vi "DASDevel.vi"() -> ()   [LabVIEW 2012]
uses:
  <vilib>/Utility/error.llb/DialogType.ctl
  SITK/Documents/SIToolkit/LabVIEW/Examples2012_4_1_0_4/Open-Close/CamHandle.vi
panel:
  out "Database OK?":bool
  in  "?":bool
  in  "Cycle Devices (Red)\nAcquisition (Blue)":bool
  in  "Image Tabs":T1(tab)
  in  "Display Image":dbl(ring) items=["2014-01-09_18;19;45", "2014-01-09_18;20;17"]
  out "Normalized Image":dbl[][](graph)
  out "Atoms":i16[][](graph)
  out "No Atoms":i16[][](graph)
  out "Dark Field":i16[][](graph)
  in  "Image Tabs 2":T1(tab)
  out "Intensity Graph":dbl[][](graph)
  out "PF Atoms":u16[][](graph)
  out "PF No Atoms":u16[][](graph)
  out "PF Dark":u16[][](graph)
  in  "Record 3":bool
  in  "bUseBuffer1 3":bool
  in  "bUseBuffer0 3":bool
  in  "Record 2":bool
  in  "bUseBuffer1 2":bool
  in  "bUseBuffer0 2":bool
  in  "bUseBuffer0":bool
  in  "bUseBuffer1":bool
  in  "Open StructureIn":T2={"Size"=88, "InterfaceType"=0, "Camera Number"=0, "CameraNumAtInterface"=0, "OpenFlags"=[], "OpenDWFlags"=[], "OpenPtrs"=[]}
  out "Bits/pixel":u16
  out "BufNr1":i16
  out "BufNr0":i16
  in  "error in (no error)":errorcluster
  in  "Camera Handle 2":u32
  in  "File and Display Name 2":string
  in  "error in (no error) 2":errorcluster
  in  "Errors":errorcluster
  in  "?":T3(tab)
  in  "Scaling":dbl(slide)=0.0016108638057548662 scale=0.001..0.1
  in  "PF Scale":dbl(slide)=0.9838778342396336 scale=0.001..10.0
  out "Elapsed Time":u32
  out "Database Output":string
  in  "ADC Gain":i32=-1 min=-1 step=1
  in  "ADC Speed":i32=-1 min=-3 step=1
  in  "Exposure (sec)":dbl format="%.3f"
  in  "Number of Images":u32=1
  in  "Number of Accumulations":u32=1
  in  "Acquire / Focus Flag":u32(ring)=2 items=["Synchronous Focus Mode"=1, "Synchronous NFrame Mode"=2, "Asynchronous Mode"=3, "Sequence Mode"=4]
  in  "Timing Mode":u32(ring)=4 items=["Free Run"=1, "Trigger First"=2, "Strobe"=3, "Bulb"=4, "Variable"=5, "Flash"=6]
  in  "Trigger Edge":u32(ring)=1 items=["Rising"=1, "Falling"=2]
  in  "Milliseconds Between Shots":u32=200
  in  "TriggerMode":u16(ring)=2 items=["Auto", "Software", "External sequence start ", "External exposure control"]
  in  "StorageMode":bool
  in  "Delay":u32=100
  in  "Exposure":u32=30
  in  "ExposureTimeBase":u16(ring)=1 items=["nanoseconds", "microseconds", "milliseconds"]
  in  "DelayTimeBase":u16(ring)=2 items=["nanoseconds", "microseconds", "milliseconds"]
  in  "ROIX0":u16=1 min=1
  in  "ROIY0":u16=1 min=1
  in  "ROIY1":u16=1 min=1
  in  "ROIX1":u16=1 min=1
  in  "Rate":i32
  in  "InterfaceType":u16(ring)=6 items=["IEEE1394 - Firewire", "IEEE1394/Firewire", "Matrox Helios Camera Link", "Silicon Software ME3 Camera Link", "National Instruments Camera Link", "Gigabit Ethernet", "USB", "Reserved", "Reserved", "Reserved", "Generic Camera Link with CLSER.DLL"]
  out "Top of Chamber Monitor":dynamicdata(graph)
  # "Stop Button"
  # "DAS Mode Select"
  # "CoolSnap HQ"
  # "PixelFly"
  # "Basic Setup"
  # "Triggering Setup"
  # "Advanced Setup"
  # "For everyday use, Number of Accumulations should be 1"
  # "Basic Setup for PixelFly"
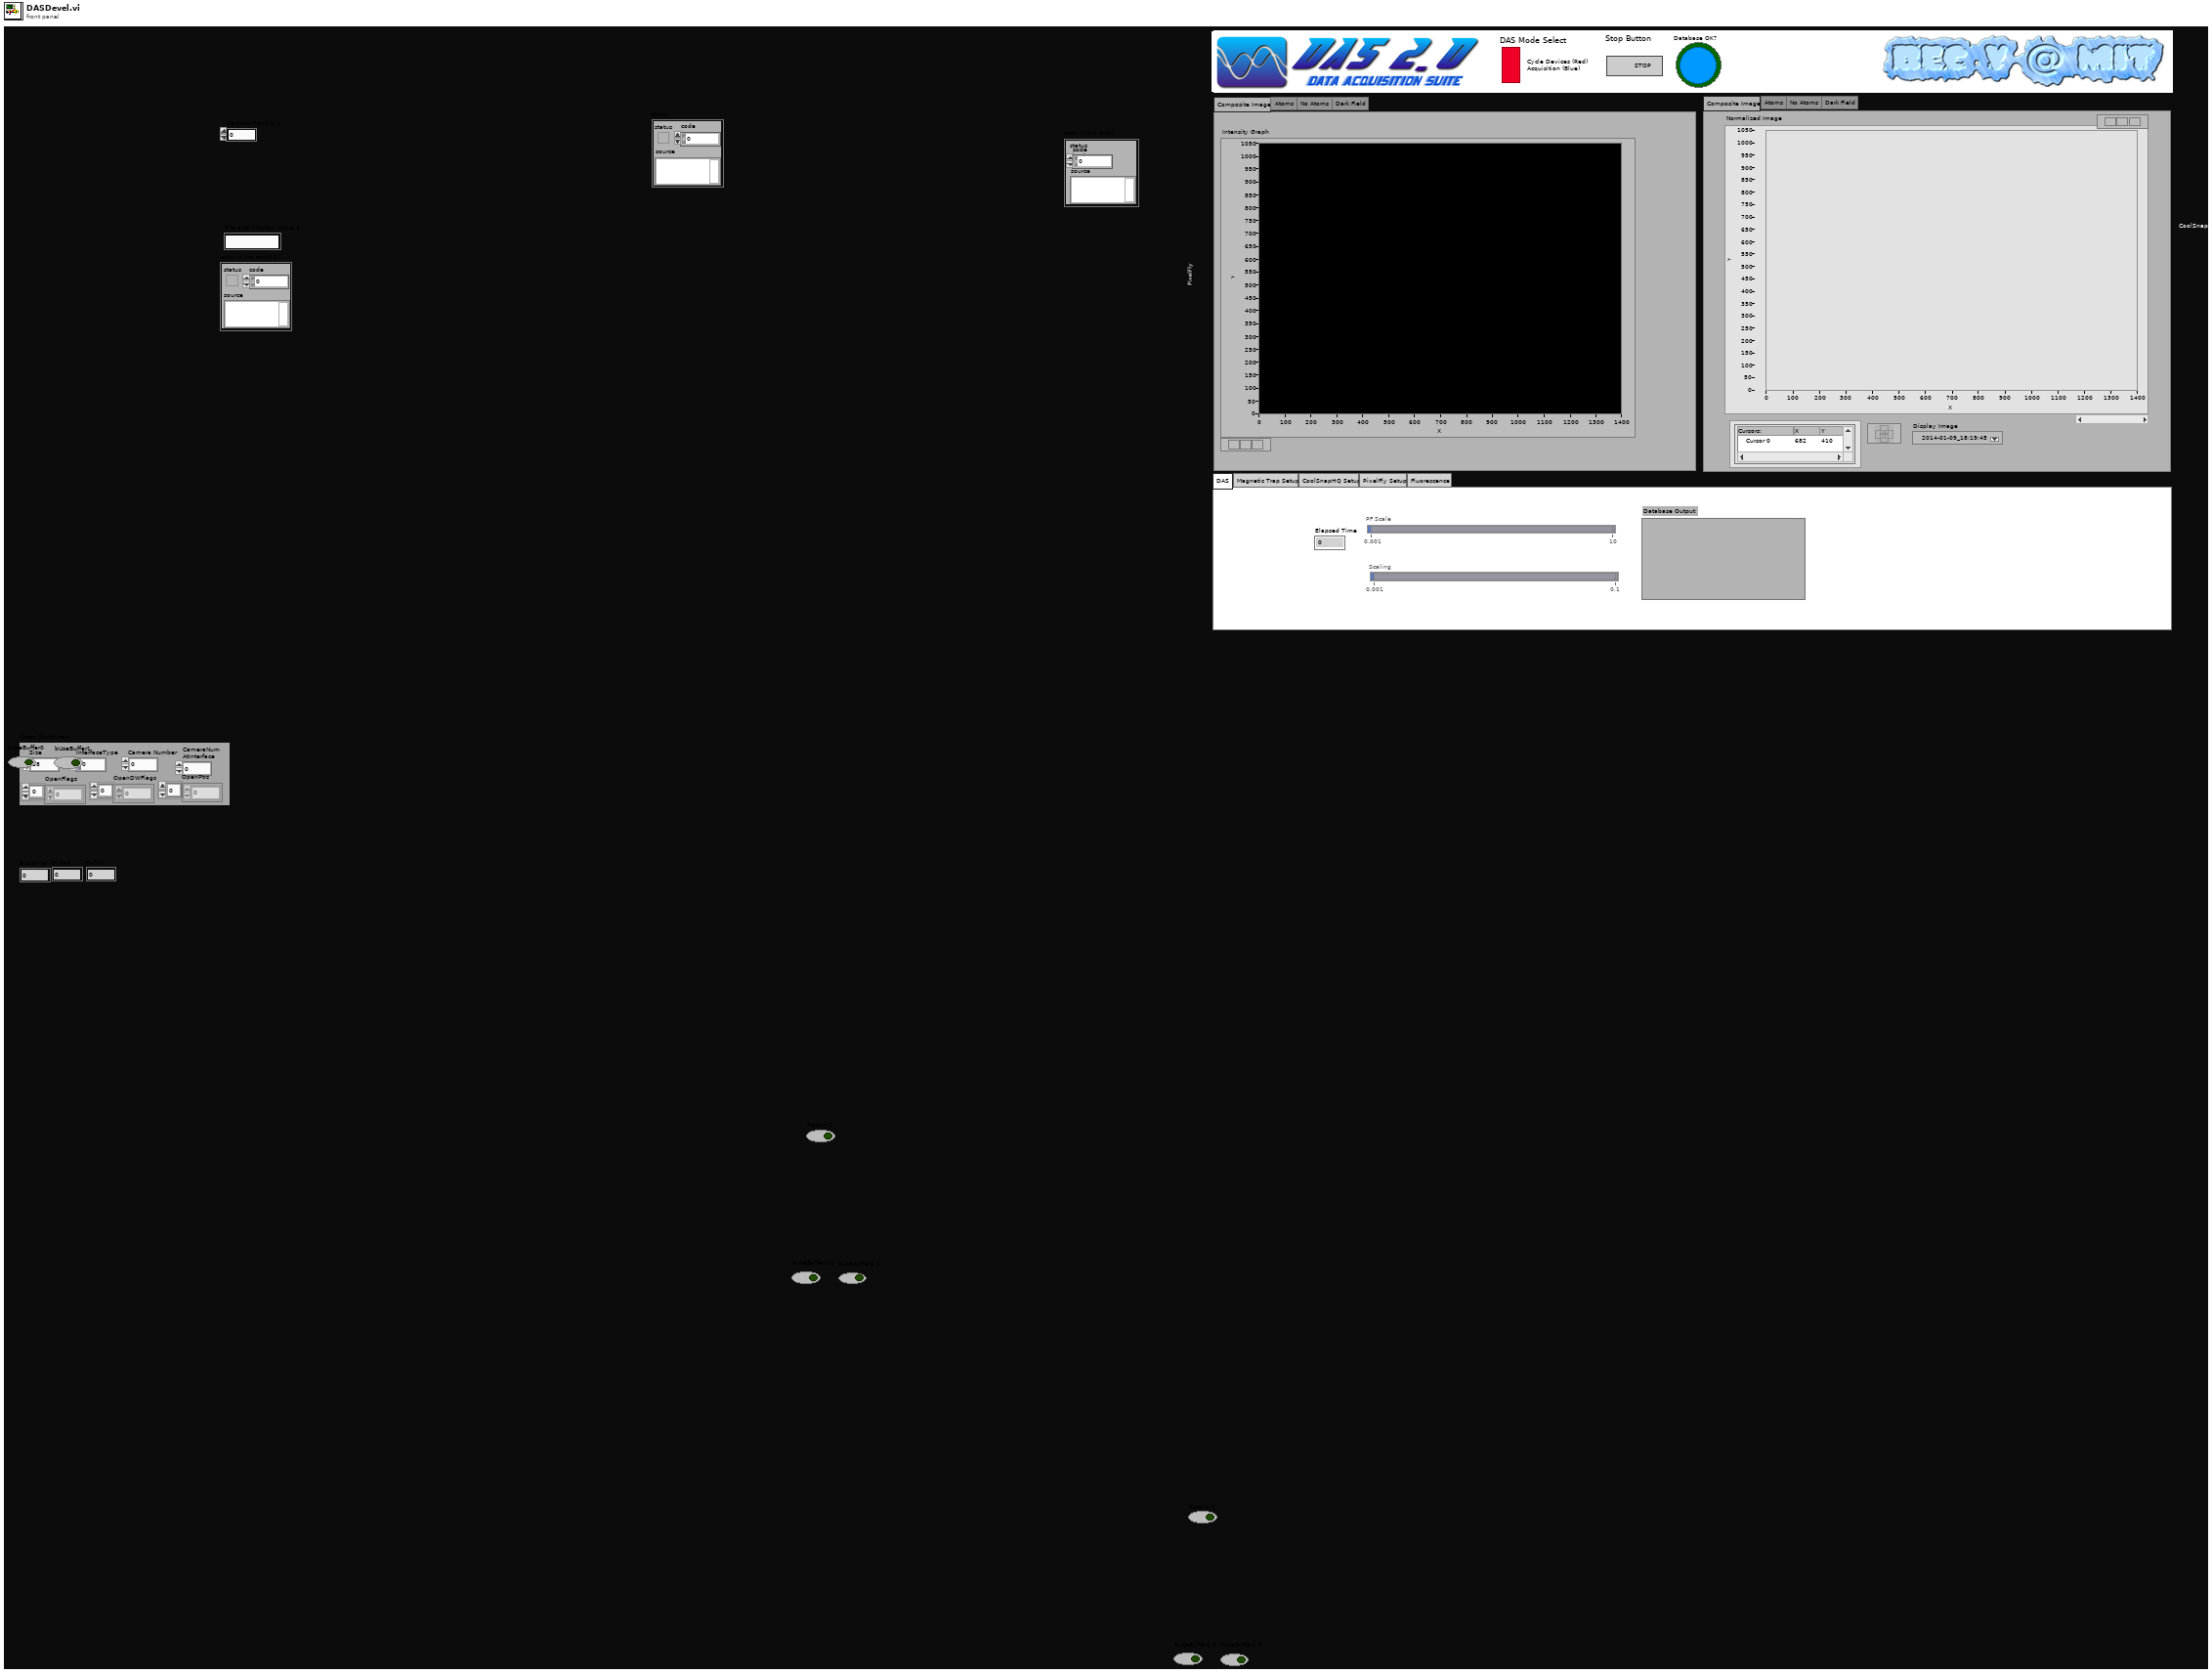
[diagram p1: front panel]
types:
  T1 = enum32{"Composite Image", "Atoms", "No Atoms", "Dark Field"}
  T2 = cluster{"Size":u16, "InterfaceType":u16, "Camera Number":u16, "CameraNumAtInterface":u16, "OpenFlags":u16[], "OpenDWFlags":u32[], "OpenPtrs":u32[]}
  T3 = enum32{"DAS", "Magnetic Trap Setup", "CoolSnapHQ Setup", "PixelFly Setup", "Fluorescence"}
  T4 = enum16{"open", "replace", "create", "open or create", "replace or create", "replace or create with confirmation"}
  T5 = enum16{"big-endian, network order", "native, host order", "little-endian"}
  T6 = typedef "DialogType.ctl" = u16
  T7 = cluster{"Size":u16, "CamType":u16, "CamSubType":u16, "SerialNumber":u32, "HWVersion":u32, "FWVersion":u32, "InterfaceType":u16, "HardwareVersion":cluster{"BoardNum":u16, "HWVersions":cluster{"BoardName":string, "BatchNumber":u16, "MinorRevision":u8, "MajorRevision":u8, "Variant":u16}[]}, "FirmwareVersion":cluster{"DeviceNum":u16, "FWVersions":cluster{"DeviceName":string, "MinorRevision":u8, "MajorRevision":u8, "Variant":u16}[]}}
  T8 = cluster{"Size":u16, "SensorTypeDESC":u16, "SensorSubtypeDESC":u16, "MaxHorizontalResStdDESC":u16, "MaxVerticalResStdDESC":u16, "MaxHorizontalResExtDESC":u16, "MaxVerticalResExtDESC":u16, "DynResDESC":u16, "MaxBinHorzDESC":u16, "BinHorzStepDESC":bool, "MaxBinVertDESC":u16, "BinVertStepDESC":bool, "ROIHorzStepDESC":u16, "ROIVertStepDESC":u16, "NumADCDESC":u16, "IRDESC":bool, "MinDelayDESC":u32, "MaxDelayDESC":u32, "MinDelayStepDESC":u32, "MinExpoDESC":u32, "MaxExpoDESC":u32, "MinExpoStepDESC":u32, "MinDelayIRDESC":u32, "MaxDelayIRDESC":u32, "MinExpoIRDESC":u32, "MaxExpoIRDESC":u32, "TimeTableDESC":bool, "DoubleImageDESC":bool, "MinCoolSetDESC":i16, "MaxCoolSetDESC":i16, "MDefaultCoolSetDESC":i16, "PowerDownModeDESC":bool, "OffsetRegDESC":bool, "ColorPattern":cluster{"UpperLeftColor":u8, "UpperRightColor":u8, "LowerLeftColor":u8, "LowerRightColor":u8}, "PatternTypeDESC":bool, "PixelRates":u32[], "CoversionFactors":u16[], "Reserved":u32[], "NoiseFilterCapable":bool, "HotPixelCapable":bool, "HotPixelWithNoiseFilter":bool, "ASCIITimeCapable":bool, "Extended Description":bool, "Get Extended":bool, "Reserved Flag 1":bool, "Reserved Flag 2":bool}
  T9 = cluster{"Camera Handle":u32, "File Handle":u32, "Display Handle":u32, "Image Handle":u32}
  T10 = cluster{u16[][], "XResAct":u16, "YResAct":u16, "BufNrOut":i16, "BufNrOut":i16, "ErrorOut":errorcluster, "hout":u64, "Bits/pixel":u16}
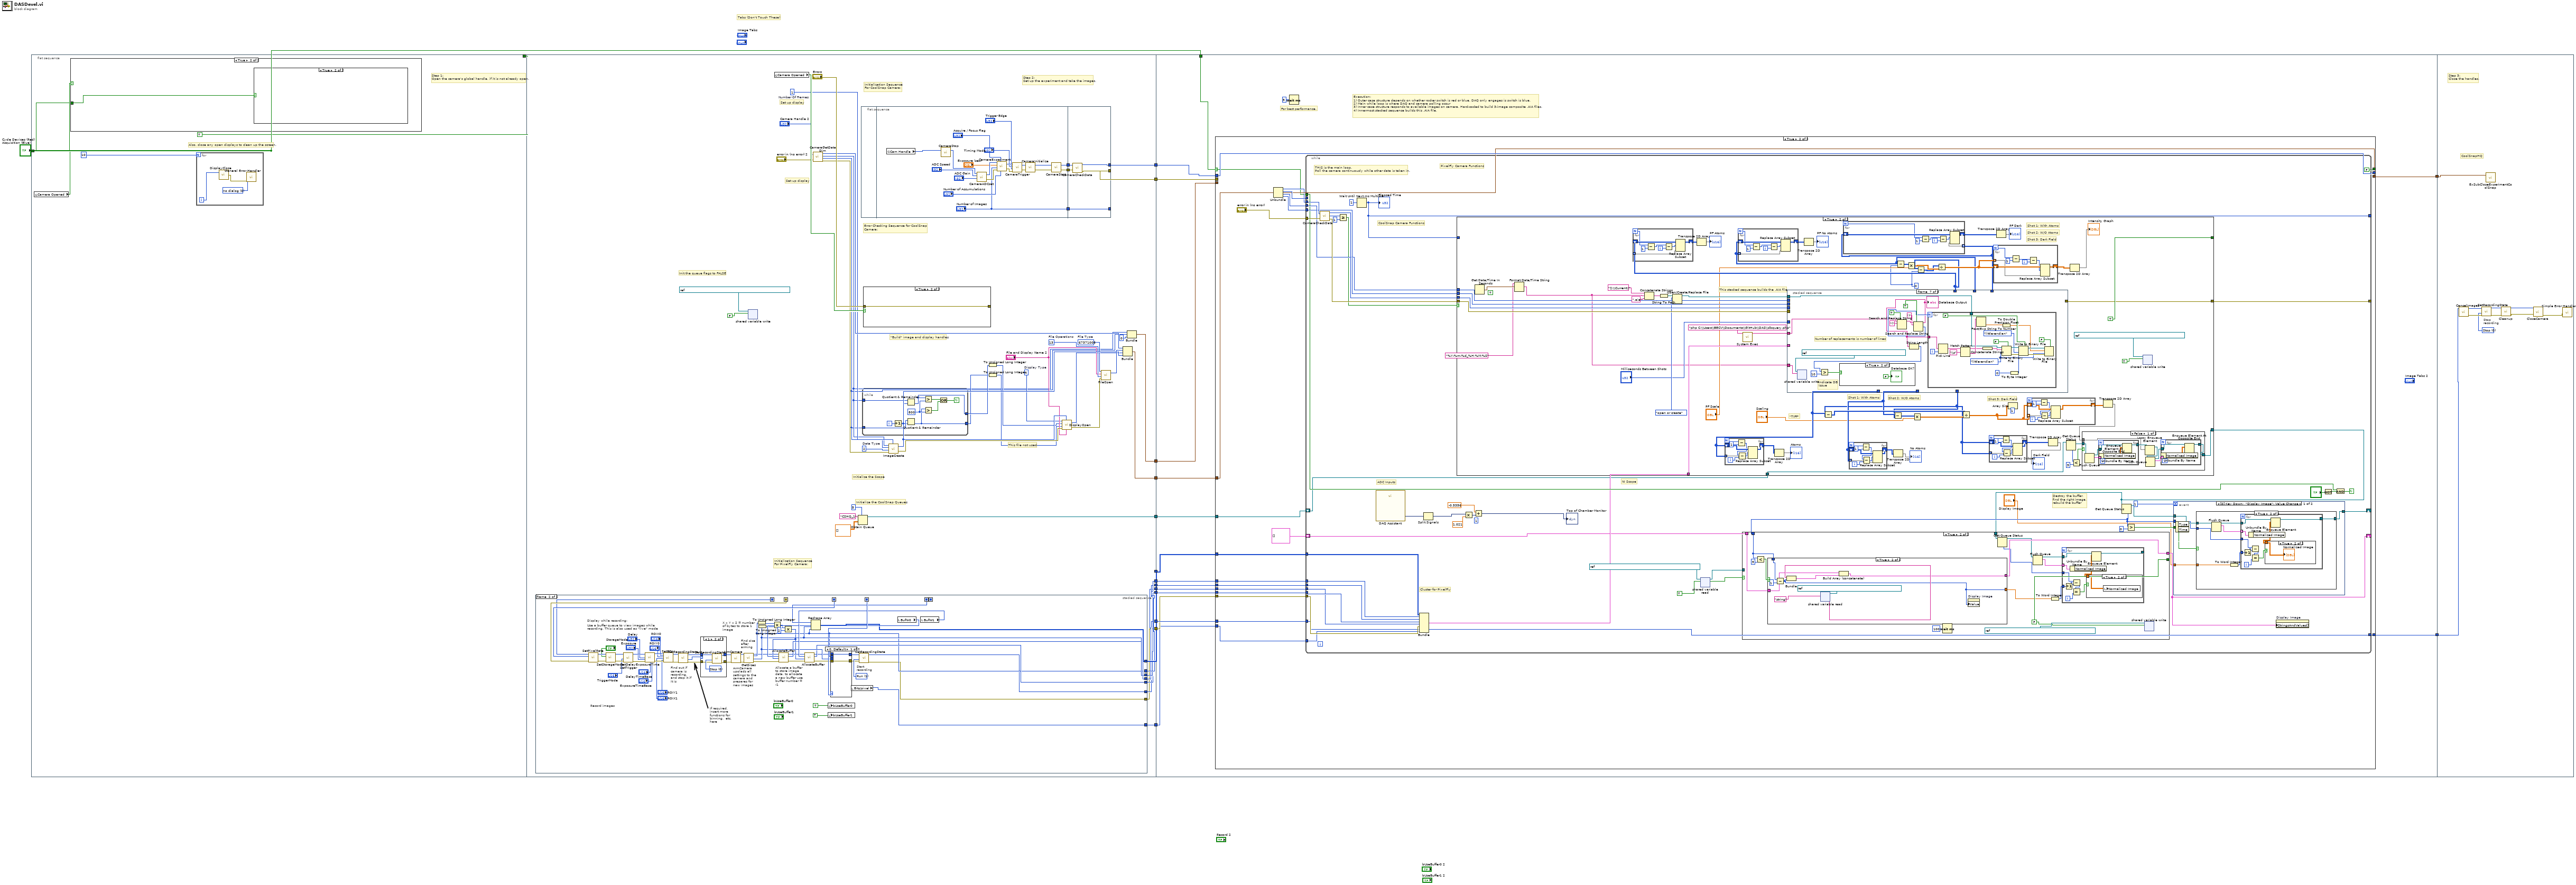
[diagram p0: block diagram]
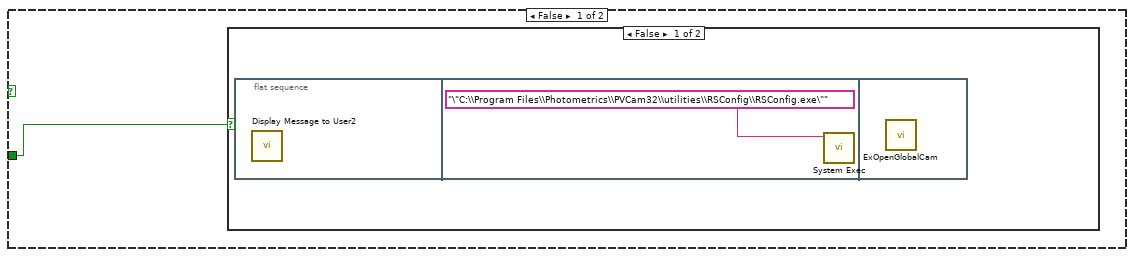
[diagram p2: hidden frame]
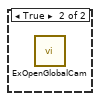
[diagram p3: hidden frame]
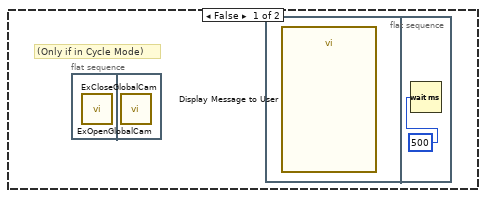
[diagram p4: hidden frame]
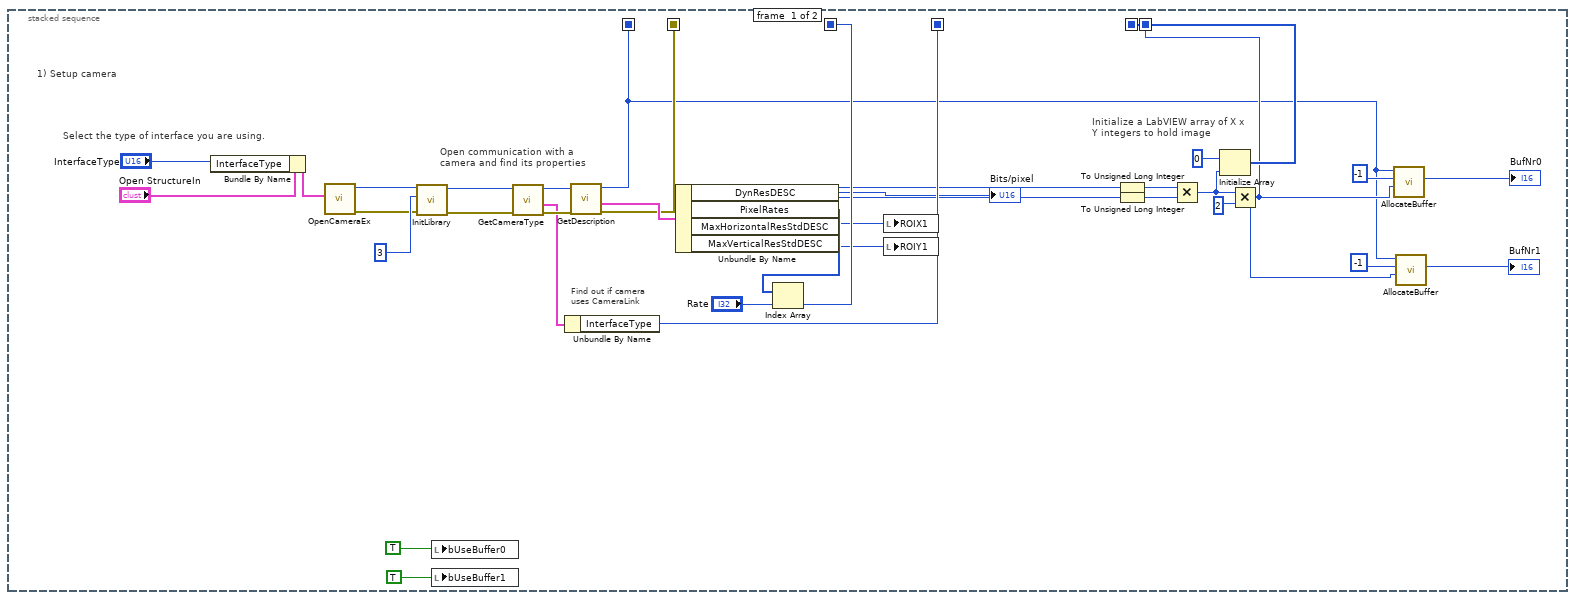
[diagram p5: hidden frame]
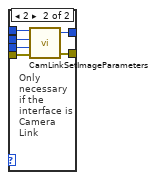
[diagram p6: hidden frame]
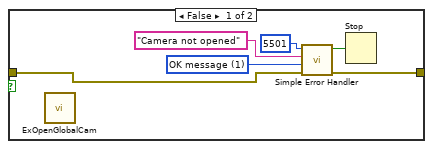
[diagram p8: hidden frame]
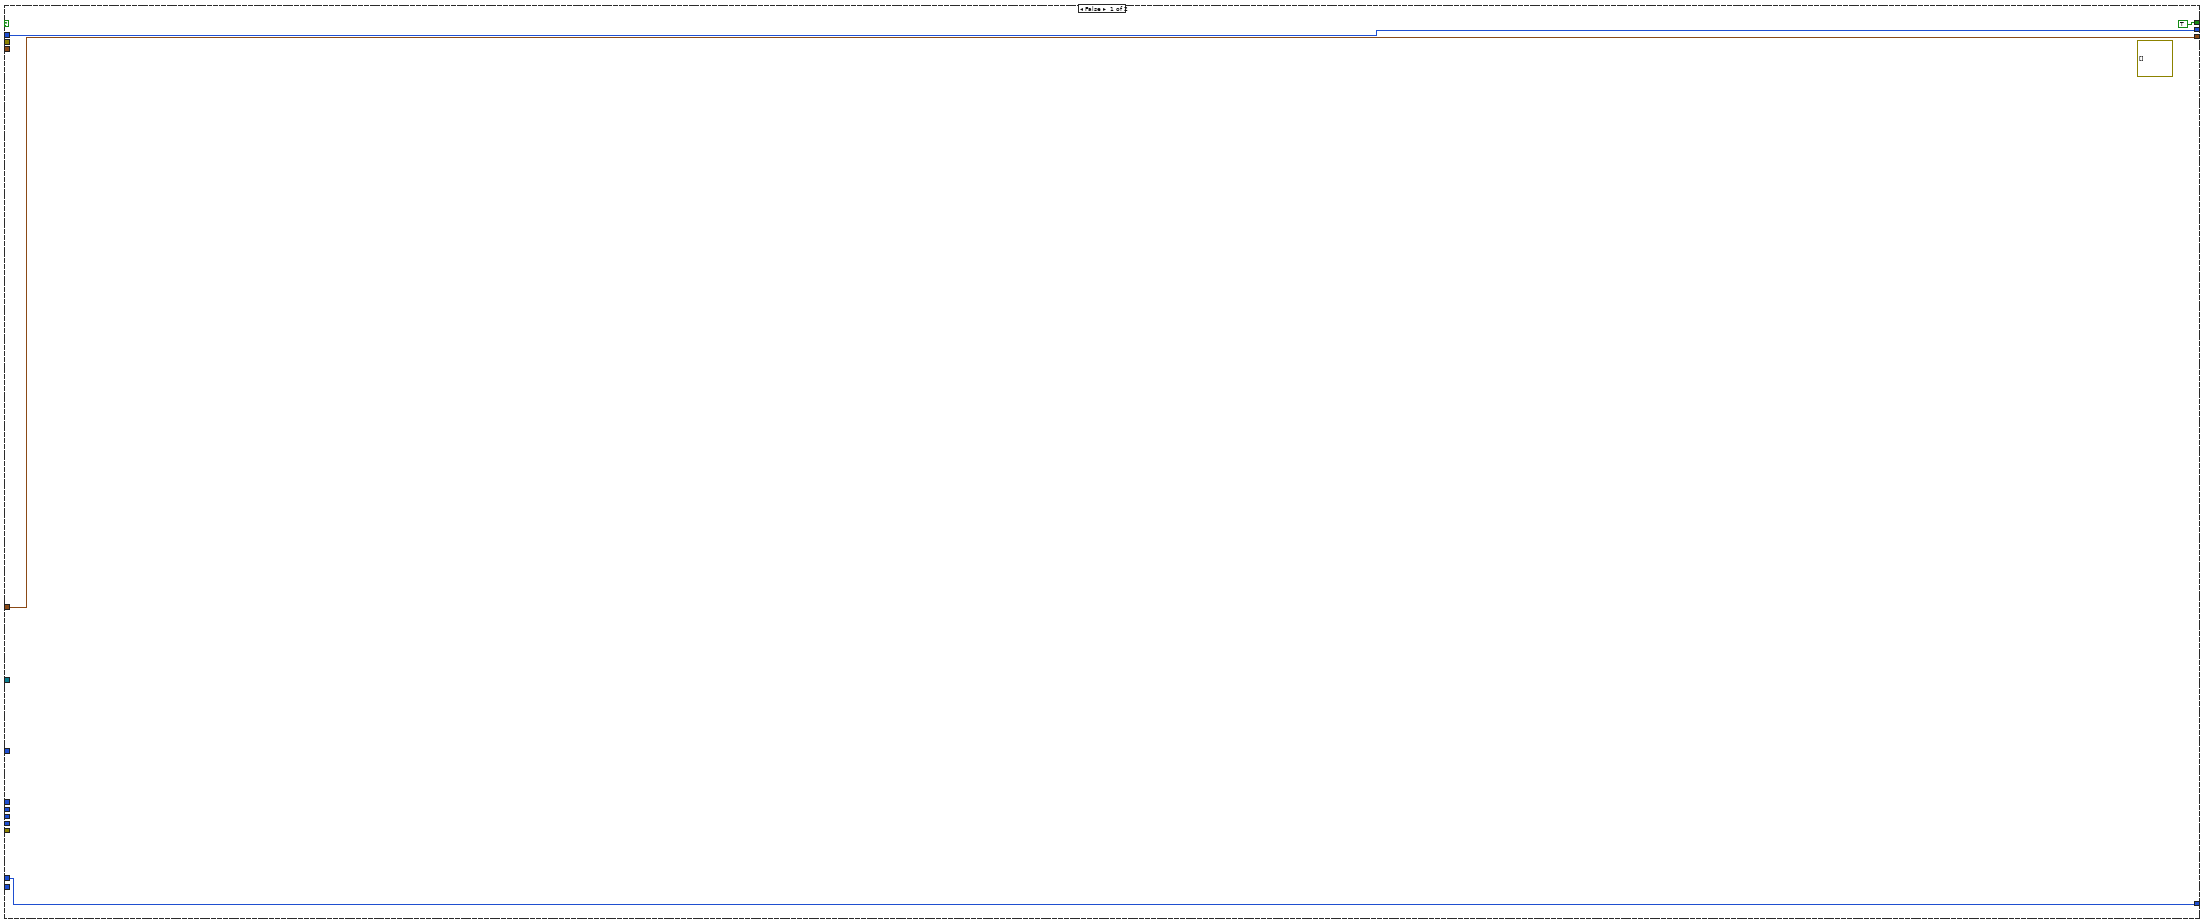
[diagram p9: hidden frame]
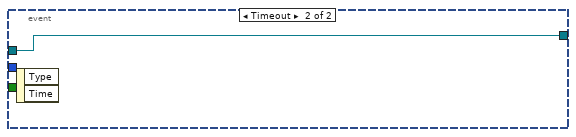
[diagram p12: hidden frame]
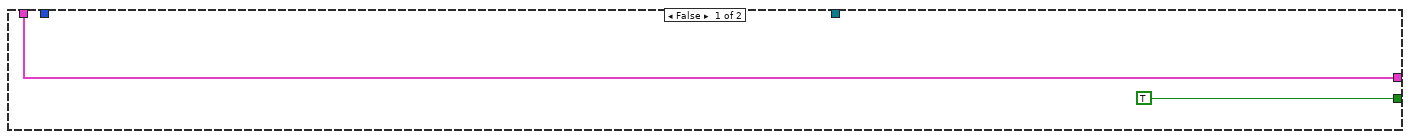
[diagram p13: hidden frame]
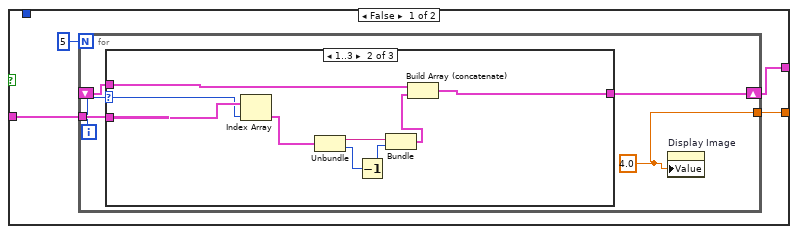
[diagram p15: hidden frame]
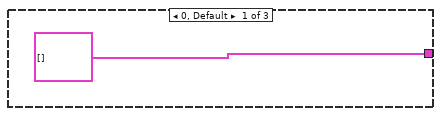
[diagram p16: hidden frame]
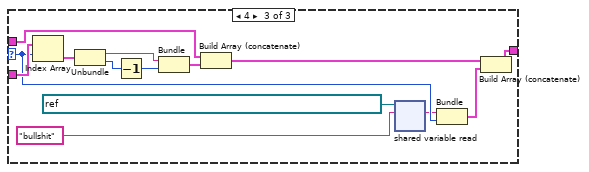
[diagram p17: hidden frame]
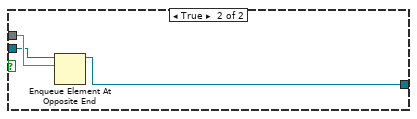
[diagram p19: hidden frame]
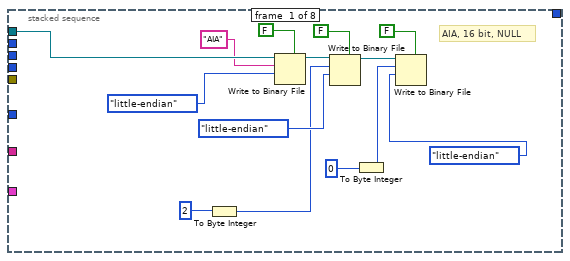
[diagram p20: hidden frame]
diagram:
  # "Tabs (Don't Touch These)"
  n1 = flat-sequence {
    tunnel: [TRUE] -> _
    tunnel: "Cycle Devices (Red)\nAcquisition (Blue)" -> [w17]
    tunnel: [w46] -> w16
    tunnel: [w45] -> w15
    tunnel: [w44] -> w14
    tunnel: [w43] -> w13
    tunnel: [w42] -> w10
    tunnel: [w41] -> w9
    tunnel: [w40] -> w8
    tunnel: [w39] -> w7
    tunnel: [w38] -> w6
    tunnel: [w37] -> w5
    tunnel: [w36] -> w4
    tunnel: [w35] -> w3
    tunnel: [w30] -> w1
    tunnel: w16 -> [w238]
    tunnel: w15 -> [w234]
    tunnel: w14 -> [w237]
    tunnel: w13 -> [w236]
    tunnel: [w235] -> w12
    tunnel: "Cycle Devices (Red)\nAcquisition (Blue)" -> [w232]
    tunnel: w10 -> [w231]
    tunnel: w9 -> [w230]
    tunnel: w8 -> [w229]
    tunnel: w7 -> [w228]
    tunnel: w6 -> [w227]
    tunnel: w5 -> [w226]
    tunnel: w4 -> [w225]
    tunnel: w3 -> [w224]
    tunnel: [w223] -> w2
    tunnel: w1 -> [w222]
    tunnel: w12 -> [w715]
    tunnel: w2 -> [w711]
    frame #0 {
      # "Also, close any open displays to clean up the screen."
      # "Step 1:\nOpen the camera's global handle, if it is not already open."
      n2 = global read "CamHandle.vi" "Camera Opened"() -> (w20:bool)
      n3 = case shown="True" w20 {
        tunnel: w17 -> [w24 w26]
        frame False {
          n4 = case shown="False" w24 {
            frame False {
              n5 = flat-sequence {
                frame #0 {
                  n6 = call "Display Message to User2"() -> ()  [unwired: 10 in, 2 out]
                }
                frame #1 {
                  n7 = call <vilib>:"System Exec.vi"("command line"="\"C:\\Program Files\\Photometrics\\PVCam32\\utilities\\RSConfig\\RSConfig.exe\"") -> ()  [unwired: 7 in, 4 out]
                }
                frame #2 {
                  n8 = call "ExOpenGlobalCam.vi"() -> ()  [unwired: 1 in]
                }
              }
            }
            frame True {
              n9 = call "ExOpenGlobalCam.vi"() -> ()  [unwired: 1 in]
            }
          }
        }
        frame True {
          n10 = case shown="True" w26 {
            frame False {
              # "(Only if in Cycle Mode)"
              n11 = flat-sequence {
                frame #0 {
                  n12 = call "ExCloseGlobalCam.vi"() -> ()  [unwired: 1 in]
                }
                frame #1 {
                  n13 = call "ExOpenGlobalCam.vi"() -> ()  [unwired: 1 in]
                }
              }
              n14 = flat-sequence {
                frame #0 {
                  n15 = call "Display Message to User"() -> ()  [unwired: 10 in, 2 out]
                }
                frame #1 {
                  n16 = Wait (ms)(milliseconds to wait=u32 500) -> ()  [unwired: 1 out]
                }
              }
            }
            frame True {
            }
          }
        }
      }
      n17 = for {
        N: 10 -> [_]
        i -> [w23]
        w21 = T6 0 items=["no dialog", "OK message", "continue or stop message", "OK message + warnings", "continue/stop + warnings"] ("type of dialog (OK msg:1)")
        n18 = call <userlib>:"DisplayClose.vi"("Display Handle"=w23) -> ("error out"=w22:errorcluster)  [unwired: 1 in]
        n19 = call <vilib>:"General Error Handler.vi"("type of dialog (OK msg:1)"=w21, "error in (no error)"=w22) -> ()  [unwired: 9 in, 5 out]
      }
    }
    frame #1 {
      w57 = u32 1  # Number Of Frames
      w58 = u32 4  # Display Type
      w59 = u32 2  # Data Type
      w61 = 13  # File Operations
      w62 = 67371008  # File Type
      # "Init the queue flags to FALSE"
      # "Initialize the CoolSnap Queues"
      # "Initialization Sequence \nFor PixelFly Camera:"
      # "Initialize the Scope"
      # "Error Checking Sequence for CoolSnap\nCamera:"
      # "Initialization Sequence \nFor CoolSnap Camera:"
      # "This file not used"
      # "\"Build\" image and display handles"
      # "Set up display"
      # "Set up display"
      # "Step 2:\nSet up the experiment and take the images."
      n20 = stacked-sequence {
        seq-local: [w103 _] -> [_ w161]
        seq-local: [w84 _] -> [_ _]
        seq-local: [w96 _] -> [_ w163]
        seq-local: [w83 _] -> [_ w158]
        seq-local: [w95 _] -> [_ w164]
        seq-local: [w94 _] -> [_ w162]
        tunnel: [_ w157] -> w42
        tunnel: [_ w153] -> w41
        tunnel: [_ w156] -> w40
        tunnel: [_ w155] -> w39
        tunnel: [_ w154] -> w38
        tunnel: [_ w152] -> w37
        tunnel: [_ w151] -> w36
        tunnel: [_ w150] -> w35
        frame #0 {
          # "Select the type of interface you are using."
          # "1) Setup camera"
          # "Find out if camera uses CameraLink"
          # "Initialize a LabVIEW array of X x Y integers to hold image"
          # "Open communication with a camera and find its properties"
          n21 = Bundle By Name(cluster="Open StructureIn", "InterfaceType"="InterfaceType") -> (w91:T2)
          n22 = call "OpenCameraEx.vi"("OpenStructureIn"=w91) -> ("error out"=w75:errorcluster, "hout"=w76:u64)  [unwired: 3 in, 2 out]
          n23 = call "InitLibrary.vi"("error in (no error)"=w75, "InterfaceType"=u32 3, "ph"=w76) -> ("error out"=w73:errorcluster, "hout"=w74:u64)  [unwired: 7 in]
          n24 = local write "bUseBuffer0"(TRUE) -> ()
          n25 = local write "bUseBuffer1"(TRUE) -> ()
          n26 = call "GetCameraType.vi"("ph"=w74, "error in (no error)"=w73) -> ("hout"=w100:u64, "CameraType"=w98:T7, "error out"=w99:errorcluster)  [unwired: 1 in, 1 out]
          n27 = Unbundle By Name(w98) -> ("InterfaceType"=w94:u16)
          n28 = call "GetDescription.vi"("ErrorIn"=w99, "ph"=w100) -> ("ErrorOut"=w95:errorcluster, "Description"=w102:T8, "hout"=w83:u64)  [unwired: 2 in, 1 out]
          n29 = Unbundle By Name(w102) -> ("DynResDESC"=→"Bits/pixel":u16, "PixelRates"=w97:u32[], "MaxHorizontalResStdDESC"=w89:u16, "MaxVerticalResStdDESC"=w88:u16)
          n30 = Index Array(array=w97, index="Rate") -> (element=w96:u32)
          n31 = local write "ROIX1"(w89) -> ()
          n32 = local write "ROIY1"(w88) -> ()
          n33 = To Unsigned Long Integer(number=w89) -> (unsigned 32bit integer=w86:u32)
          n34 = To Unsigned Long Integer(number=w88) -> (unsigned 32bit integer=w85:u32)
          n35 = Multiply(x=w86, y=w85) -> (x*y=w104:u32)
          n36 = Initialize Array(u16 0 ("Element Data"), w104) -> (w103:u16[])
          n37 = Multiply(x=w104, y=u32 2) -> (x*y=w84:u32)
          n38 = call "AllocateBuffer.vi"("Size"=w84, "BufNr"=i16 -1, "ph"=w83) -> ("BufNrOut"=→"BufNr0":i16)  [unwired: 3 in, 5 out]
          n39 = call "AllocateBuffer.vi"("Size"=w84, "BufNr"=-1, "ph"=w83) -> ("BufNrOut"=→"BufNr1":i16)  [unwired: 3 in, 5 out]
        }
        frame #1 {
          w149 = u16 1 items=["Stop", "Run"] ("RecordingState")
          # "Record images"
          # "Start recording"
          # "Allocate a buffer to store image data. to allocate a new buffer use buffer number = -1"
          # "Find size after arming"
          # "ArmCamera upolads all settings to the camera and prepares for new images"
          # "Find out if camera is recording, and stop it if it is"
          # "If required, insert more functions for binning.  etc. here"
          # "X x Y x 2 = number of bytes to store 1 image"
          # "Use a buffer queue to view images while recording. This is also used as \"live\" mode"
          # "Display while recording:"
          n40 = call "SetPixelRate.vi"("error in (no error)"=w164, "PixelRate"=w163, "ph"=w158) -> ("error out"=w147:errorcluster, "hout"=w148:u64)  [unwired: 2 in, 1 out]
          n41 = call "SetStorageMode.vi"("error in (no error)"=w147, "StorageMode"="StorageMode", "ph"=w148) -> ("error out"=w139:errorcluster, "hout"=w140:u64)  [unwired: 2 in, 1 out]
          n42 = call "SetTrigger.vi"("error in (no error)"=w139, "TriggerMode"="TriggerMode", "ph"=w140) -> ("error out"=w132:errorcluster, "hout"=w133:u64)  [unwired: 2 in, 1 out]
          n43 = call "SetDelayExposureTime.vi"("ph"=w133, "Delay"="Delay", "Exposure"="Exposure", "error in (no error)"=w132, "DelayTimeBase"="DelayTimeBase", "ExposureTimeBase"="ExposureTimeBase") -> ("hout"=w121:u64, "error out"=w119:errorcluster)  [unwired: 7 in, 1 out]
          n44 = call "SetROI.vi"("ph"=w121, "ROIX0"="ROIX0", "ROIY0"="ROIY0", "ROIX1"="ROIX1", "ROIY1"="ROIY1", "error in (no error)"=w119) -> ("hout"=w120:u64, "error out"=w118:errorcluster)  [unwired: 12 in]
          n45 = call "GetRecordingState.vi"("ErrorIn"=w118, "ph"=w120) -> ("ErrorOut"=w143:errorcluster, "RecordingState"=w145:u16, "hout"=w144:u64)  [unwired: 2 in, 1 out]
          n46 = case shown="1" w145 {
            tunnel: w144 -> [w174 w178]
            tunnel: w143 -> [w173 w177]
            tunnel: [w174 w176] -> w142
            tunnel: [w173 w175] -> w141
            frame 0, Default {
            }
            frame 1 {
              w179 = u16 0 items=["Stop", "Run"] ("RecordingState")
              n47 = call "SetRecordingState.vi"("ErrorIn"=w177, "RecordingState"=w179, "ph"=w178) -> ("ErrorOut"=w175:errorcluster, "hout"=w176:u64)  [unwired: 2 in, 1 out]
            }
          }
          n48 = call "ArmCamera.vi"("error in (no error)"=w141, "ph"=w142) -> ("error out"=w137:errorcluster, "hout"=w138:u64)  [unwired: 1 in, 1 out]
          n49 = call "GetSizes.vi"("ph"=w138, "ErrorIn"=w137) -> ("hout"=w134:u64, "XResAct"=w153:u16, "YResAct"=w156:u16, "ErrorOut"=w136:errorcluster)  [unwired: 11 in, 3 out]
          n50 = To Unsigned Long Integer(number=w153) -> (unsigned 32bit integer=w122:u32)
          n51 = To Unsigned Long Integer(number=w156) -> (unsigned 32bit integer=w123:u32)
          n52 = Multiply(x=w122, y=w123) -> (x*y=w124:u32)
          n53 = Multiply(x=w124, y=u32 2) -> (x*y=w109:u32)
          n54 = Reshape Array(w161, w156, w153) -> (w157:u16[][])
          n55 = local write "bUseBuffer0"(TRUE) -> ()
          n56 = local write "bUseBuffer1"(TRUE) -> ()
          n57 = local read "Bits/pixel"() -> (w150:u16)
          n58 = local read "BufNr0"() -> (w159:i16)
          n59 = call "AllocateBuffer.vi"("error in (no error)"=w136, "Size"=w109, "BufNr"=w159, "ph"=w134) -> ("error out"=w113:errorcluster, "BufNrOut"=w155:i16, "hout"=w111:u64)  [unwired: 2 in, 3 out]
          n60 = local read "BufNr1"() -> (w160:i16)
          n61 = call "AllocateBuffer.vi"("error in (no error)"=w113, "Size"=w109, "BufNr"=w160, "ph"=w111) -> ("error out"=w112:errorcluster, "BufNrOut"=w154:i16, "hout"=w110:u64)  [unwired: 2 in, 3 out]
          n62 = case shown="0, Default" w162 {
            tunnel: w112 -> [w165 w172]
            tunnel: [w165 w171] -> w127
            tunnel: w110 -> [w166 w170]
            tunnel: [w166 w169] -> w126
            tunnel: w156 -> [_ w168]
            tunnel: w153 -> [_ w167]
            frame 0, Default {
            }
            frame 2 {
              # "Only necessary if the interface is Camera Link"
              n63 = call "CamLinkSetImageParameters.vi"("error in (no error)"=w172, "YRes"=w168, "XRes"=w167, "ph"=w170) -> ("error out"=w171:errorcluster, "hout"=w169:u64)  [unwired: 1 out]
            }
          }
          n64 = call "SetRecordingState.vi"("ErrorIn"=w127, "RecordingState"=w149, "ph"=w126) -> ("ErrorOut"=w151:errorcluster, "hout"=w152:u64)  [unwired: 2 in, 1 out]
        }
      }
      n65 = shared-variable-write(refnum<k21> "ni.var.psp://my computer/Untitled Library 1/CSHQ_1_Changed" ("shared variable refnum in"), FALSE) -> ()  [unwired: 1 in, 2 out]
      n66 = global read "CamHandle.vi" "Camera Opened"() -> (w72:bool)
      n67 = call <userlib>:"CameraGetDataDim.vi"("Camera Handle"="Camera Handle 2", "error in"="error in (no error) 2") -> ("Camera Handle"=w65:u32, "Xdim"=w49:u32, "Ydim"=w48:u32, "error out"=w70:errorcluster)
      n68 = Obtain Queue(max queue size (-1, unlimited)=5, name (unnamed)="CSHQ_1", element data type=dbl[][] [] ("Normalized Image")) -> (queue out=w30:refnum<queue>)  [unwired: 2 in, 2 out]
      n69 = flat-sequence {
        tunnel: ["Number of Images"] -> w52
        tunnel: [w186] -> w51
        tunnel: [w185] -> w50
        tunnel: [w200] -> w44
        tunnel: [w204] -> _
        tunnel: w52 -> [w204]
        tunnel: w51 -> [w203]
        tunnel: w50 -> [w202]
        tunnel: [w201] -> w43
        frame #0 {
        }
        frame #1 {
          n70 = global read "CamHandle.vi" "Cam Handle"() -> (w180:u32)
          n71 = call <userlib>:"CameraStop.vi"("Camera Handle"=w180) -> ("Camera Handle"=w181:u32)  [unwired: 1 in, 1 out]
          n72 = call <userlib>:"CameraADCset.vi"("ADC Gain"="ADC Gain", "ADC Speed"="ADC Speed", "Camera Handle"=w181) -> ("error out"=w197:errorcluster, "Camera Handle"=w199:u32)  [unwired: 3 in]
          n73 = call <userlib>:"CameraExperiment.vi"("Number of Accumulations"="Number of Accumulations", "Acquire / Focus Flag"="Acquire / Focus Flag", "error in"=w197, "Number of Images"="Number of Images", "Exposure (sec)"="Exposure (sec)", "Camera Handle"=w199) -> ("error out"=w191:errorcluster, "Camera Handle"=w192:u32)
          n74 = call <userlib>:"CameraTrigger.vi"("error in"=w191, "Trigger Edge"="Trigger Edge", "Timing Mode"="Timing Mode", "Camera Handle"=w192) -> ("error out"=w182:errorcluster, "Camera Handle"=w187:u32)
          n75 = call <userlib>:"CameraInitialize.vi"("error in"=w182, "Camera Handle"=w187) -> ("error out"=w184:errorcluster, "Camera Handle"=w183:u32)
          n76 = call <userlib>:"CameraStart.vi"("error in"=w184, "Camera Handle"=w183) -> ("error out"=w185:errorcluster, "Camera Handle"=w186:u32)
        }
        frame #2 {
          n77 = call <userlib>:"CameraCheckData.vi"("Camera Handle"=w203, "error in"=w202) -> ("Camera Handle"=w200:u32, "error out"=w201:errorcluster)  [unwired: 1 out]
        }
      }
      n78 = while {
        tunnel: w49 -> [w213]
        tunnel: w48 -> [w212]
        tunnel: [w207] -> w56
        tunnel: [w206] -> w55
        i -> [w211]
        stop <- w208 continue-if-true
        w214 = 800
        n79 = Increment(x=w211) -> (x+1=w205:i32)
        n80 = Quotient & Remainder(x=w213, y=w205) -> (floor(x/y)=w207:u32)  [unwired: 1 out]
        n81 = Quotient & Remainder(x=w212, y=w205) -> (floor(x/y)=w206:u32)  [unwired: 1 out]
        n82 = Greater?(x=w207, y=w214) -> (0:w210:bool)
        n83 = Greater?(x=w206, y=w214) -> (0:w209:bool)
        n84 = Or(x=w210, y=w209) -> (x .or. y?=w208:bool)
      }
      n85 = case shown="True" w72 {
        tunnel: [w219 w221] -> _
        tunnel: "Errors" -> [w215 w221]
        frame False {
          w220 = u16 1 items=["no dialog", "OK message", "continue or stop message"] ("type of dialog (OK msg:1)")
          n86 = call "ExOpenGlobalCam.vi"() -> ()  [unwired: 1 in]
          n87 = call <vilib>:"Simple Error Handler.vi"("error code (no error:0)"=5501, "error source (\" \")"="Camera not opened", "type of dialog (OK msg:1)"=w220, "error in (no error)"=w215) -> ("error?"=w217:bool, "error out"=w219:errorcluster)  [unwired: 1 in, 3 out]
          n88 = Stop(stop? (T)=w217) -> ()
        }
        frame True {
        }
      }
      n89 = call <userlib>:"ImageCreate.vi"("X dimension"=w49, "Y dimension"=w48, "Data Type"=w59, "error in"=w70, "Number Of Frames"=w57) -> ("Image Handle"=w63:u32, "error out"=w69:errorcluster)
      n90 = To Unsigned Long Integer(number=w56) -> (unsigned 32bit integer=w54:u32)
      n91 = To Unsigned Long Integer(number=w55) -> (unsigned 32bit integer=w53:u32)
      n92 = call <userlib>:"DisplayOpen.vi"("Display Title"="File and Display Name 2", "Image Handle"=w63, "error in"=w69, "Display Height"=w53, "Display Width"=w54, "Display Type"=w58) -> ("error out"=w68:errorcluster, "Display Handle"=w34:u32)
      n93 = call <userlib>:"FileOpen.vi"("error in"=w68, "File Operations"=w61, "FileName"="File and Display Name 2", "File Type"=w62) -> ("File Handle"=w64:u32)  [unwired: 1 out]
      n94 = Bundle("Camera Handle"=w65, "File Handle"=w64, "Display Handle"=w34, "Image Handle"=w63) -> (w45:T9)  [unwired: 1 in]
      n95 = Bundle("Xdim"=w49, "Ydim"=w48, 0) -> (w46:cluster{"Xdim":u32, "Ydim":u32, i32})  [unwired: 1 in]
    }
    frame #2 {
      # "For best performance."
      # "Execution:\n1) Outer case structure depends on whether rocker switch is red or blue. DAQ only engages is switch is blue.\n2) Main while loop is where DAQ and camera polling occur\n3) Inner case structure responds to available images on camera. Hard-coded to build 3-image composite .AIA files.\n4) Innermost stacked sequence builds this .AIA file."
      n96 = case shown="True" w232 {
        selector: w232 -> [_ w254]
        tunnel: w234 -> [w242 w256]
        tunnel: [w242 w256] -> w235
        tunnel: w237 -> [w241 w261]
        tunnel: w236 -> [_ _]
        tunnel: [w241 w261] -> _
        tunnel: [TRUE FALSE] -> _
        tunnel: w238 -> [_ _]
        tunnel: w231 -> [_ w253]
        tunnel: w230 -> [_ w252]
        tunnel: w229 -> [_ w251]
        tunnel: w228 -> [_ w250]
        tunnel: w227 -> [_ w249]
        tunnel: w226 -> [w239 w248]
        tunnel: w225 -> [_ w247]
        tunnel: w224 -> [_ w246]
        tunnel: [w239 w245] -> w223
        tunnel: w222 -> [_ w244]
        frame False {
          (unwired) errorcluster[] []
        }
        frame True {
          n97 = Unbundle(w256) -> ("Camera Handle"=w255:u32, "File Handle"=w259:u32, "Display Handle"=w258:u32, "Image Handle"=w257:u32)
          n98 = while {
            tunnel: "error in (no error)" -> [w308]
            tunnel: w255 -> [w307]
            tunnel: [w304] -> _
            tunnel: w259 -> [_]
            tunnel: w258 -> [w303]
            tunnel: w257 -> [w302]
            tunnel: [w300] -> _
            tunnel: w254 -> [w290]
            tunnel: w253 -> [w286]
            tunnel: w252 -> [w285]
            tunnel: w251 -> [w284]
            tunnel: w250 -> [w282]
            tunnel: w249 -> [w283]
            tunnel: w248 -> [w278]
            tunnel: w247 -> [w281]
            tunnel: w246 -> [w280]
            tunnel: [w278] -> w245
            shift-right: [w277] -> _
            shift-left: w244 -> [w264]
            shift-right: [w270] -> _
            shift-left: cluster{"date/time string":string, i32}[] [] -> [w271]
            stop <- w289 continue-if-true
            (unwired) 1
            # "Destroy the buffer,\nfind the right image,\nrebuild the buffer"
            # "Cluster for PixelFly"
            # "PixelFly Camera Functions"
            # "NI Scope"
            # "CoolSnap Camera Functions"
            # "ADC Inputs"
            # "THIS is the main loop.\nPoll the camera continuously while other data is taken in."
            n99 = call <userlib>:"CameraCheckData.vi"("Camera Handle"=w307, "error in"=w308) -> ("Camera Handle"=w306:u32, "Number Of Frames Available"=w299:i32, "error out"=w305:errorcluster)
            n100 = Greater Or Equal?(x=w299, y=1) -> (x >= y?=w297:bool)
            n101 = Wait Until Next ms Multiple(millisecond multiple=1) -> (millisecond timer value=w300:u32)
            "Elapsed Time" <- w300
            n102 = call "DAQ Assistant"() -> ("data"=w296:dynamicdata)  [unwired: 17 in, 2 out]
            n103 = Bundle(w286, "XResAct"=w285, "YResAct"=w284, "BufNrOut"=w283, "BufNrOut"=w282, "ErrorOut"=w281, "hout"=w278, "Bits/pixel"=w280) -> (w279:T10)  [unwired: 1 in]
            n104 = Split Signals(w296) -> (w295:dynamicdata)  [unwired: 3 in, 2 out]
            n105 = case shown="True" w297 {
              selector: w297 -> [w405 _]
              tunnel: w306 -> [_ w466]
              tunnel: w305 -> [w406 w465]
              tunnel: [w405 TRUE] -> _
              tunnel: [w406 w455] -> w304
              tunnel: w303 -> [_ w464]
              tunnel: w302 -> [_ w461]
              tunnel: w300 -> [_ _]
              tunnel: w279 -> [_ w446]
              tunnel: w264 -> [w404 w415]
              tunnel: [w404 w412] -> w263
              frame False {
              }
              frame True {
                w419 = 0 ("y")
                (unwired) 1 ("index")
                (unwired) TRUE ("want seconds? (F)")
                # "Shot 1: With Atoms"
                # "Shot 3: Dark Field"
                # "Shot 2: W/O Atoms"
                # "Shot 3: Dark Field"
                # "Shot 2: W/O Atoms"
                # "Shot 1: With Atoms"
                # "This stacked sequence builds the .AIA file"
                # "\"TIFF\""
                n106 = Get Date/Time In Seconds() -> (seconds since 1Jan1904=w448:timestamp)
                n107 = Format Date/Time String(time format string (%c)="%Y-%m-%d_%H;%M;%S", seconds (now)=w448) -> (date/time string=w409:string)  [unwired: 1 in]
                n108 = Concatenate Strings("Z:\\Current\\" ("string"), w409, ".aia" ("string")) -> (w459:string)
                n109 = String To Path(string=w459) -> (path=w458:path)
                n110 = Open/Create/Replace File(file path (use dialog)=w458, operation (0:open)=T4."open or create") -> (refnum out=w457:refnum<file>)  [unwired: 4 in, 2 out]
                n111 = call <vilib>:"System Exec.vi"("command line"="php C:\\Users\\BECV\\Documents\\GitHub\\DAS\\dbquery.php") -> ("standard output"=w407:string)  [unwired: 7 in, 3 out]
                n112 = stacked-sequence {
                  tunnel: w466 -> [_ w604 _ w637 _ w667 _ _]
                  tunnel: w465 -> [_ _ _ _ _ _ _ _]
                  tunnel: w464 -> [_ w606 _ w634 _ w664 _ _]
                  tunnel: w461 -> [_ w605 _ w633 _ w663 _ _]
                  tunnel: w457 -> [w564 w598 _ w635 _ w665 w676 w705]
                  tunnel: [_ w601 _ _ _ _ _ _] -> w455
                  tunnel: "Milliseconds Between Shots" -> [_ _ w608 _ w638 _ _ _]
                  tunnel: [_ w582 _ _ _ _ _ _] -> w443
                  tunnel: [_ _ _ w629 _ _ _ _] -> w438
                  tunnel: [_ _ _ _ _ w659 _ _] -> w437
                  tunnel: w446 -> [_ w566 _ w613 _ w643 _ _]
                  tunnel: [_ w565 _ _ _ _ _ _] -> w434
                  tunnel: [_ _ _ w612 _ _ _ _] -> w431
                  tunnel: [_ _ _ _ _ w642 _ _] -> w428
                  tunnel: w409 -> [_ _ _ _ _ _ w673 _]
                  tunnel: w407 -> [_ _ _ _ _ _ w668 _]
                  frame #0 {
                    # "AIA, 16 bit, NULL"
                    n113 = To Byte Integer(number=2) -> (8bit integer=w553:i8)
                    n114 = Write to Binary File(file (use dialog)=w564, data="AIA", 5:FALSE ("prepend array or string size? (T)"), 9:T5."little-endian" ("byte order (0:big-endian, network order)")) -> (refnum out=w560:refnum<file>)  [unwired: 2 in, 2 out]
                    n115 = Write to Binary File(file (use dialog)=w560, data=w553, 5:FALSE ("prepend array or string size? (T)"), 9:T5."little-endian" ("byte order (0:big-endian, network order)")) -> (refnum out=w559:refnum<file>)  [unwired: 2 in, 2 out]
                    n116 = To Byte Integer(number=0) -> (8bit integer=w551:i8)
                    n117 = Write to Binary File(file (use dialog)=w559, data=w551, 5:FALSE ("prepend array or string size? (T)"), 9:T5."little-endian" ("byte order (0:big-endian, network order)")) -> ()  [unwired: 2 in, 3 out]
                  }
                  frame #1 {
                    w577 = 0
                    w591 = T5."little-endian" ("byte order (0:big-endian, network order)")
                    n118 = call <userlib>:"CameraGetData.vi"("Data Handle"=w605, "Camera Handle"=w604) -> ("error out"=w607:errorcluster, "Data Handle"=w602:u32)  [unwired: 1 in, 1 out]
                    n119 = To Word Integer(number=3 ("index")) -> (16bit integer=w586:i16)
                    n120 = call <userlib>:"ImageGetArrayI32.vi"("Image Handle"=w602) -> ("Array int 32"=w583:i32[][])  [unwired: 2 in, 2 out]
                    n121 = call <userlib>:"DisplayImage.vi"("error in"=w607, "Image Handle"=w602, "Display Handle"=w606) -> ()  [unwired: 1 in, 2 out]
                    n122 = Array Size(array=w583) -> (size(s)=w584:i32[])
                    n123 = Index Array(array=w584, index=1) -> (element=w588:i32)
                    n124 = Index Array(array=w584, index=0) -> (element=w589:i32)
                    n125 = To Word Integer(number=w583) -> (16bit integer=w582:i16[][])
                    n126 = To Word Integer(number=w589) -> (16bit integer=w590:i16)
                    n127 = To Word Integer(number=w588) -> (16bit integer=w587:i16)
                    n128 = Write to Binary File(file (use dialog)=w598, data=w590, 5:FALSE ("prepend array or string size? (T)"), 9:w591) -> (refnum out=w597:refnum<file>)  [unwired: 2 in, 2 out]
                    n129 = Write to Binary File(file (use dialog)=w597, data=w587, 5:FALSE ("prepend array or string size? (T)"), 9:w591) -> (refnum out=w596:refnum<file>)  [unwired: 2 in, 2 out]
                    n130 = Write to Binary File(file (use dialog)=w596, data=w586, 5:FALSE ("prepend array or string size? (T)"), 9:w591) -> (refnum out=w595:refnum<file>)  [unwired: 2 in, 2 out]
                    n131 = Write to Binary File(file (use dialog)=w595, data=w582, 5:FALSE ("prepend array or string size? (T)"), 9:w591) -> (error out=w601:errorcluster)  [unwired: 2 in, 2 out]
                    n132 = Unbundle(w566) -> (w574:u16[][], "XResAct"=w573:u16, "YResAct"=w572:u16, "BufNrOut"=w571:i16, "BufNrOut"=w570:i16, "ErrorOut"=w569:errorcluster, "hout"=w568:u64, "Bits/pixel"=w567:u16)
                    n133 = call "AddBufferEX.vi"("ph"=w568, "BuffNr"=i16 0, "1stImage"=w577, "LastImage"=w577, "error in (no error)"=w569, "XRes"=w573, "YRes"=w572, "BitPerPixel"=w567) -> ("hout"=w579:u64, "error out"=w578:errorcluster)  [unwired: 5 in, 1 out]
                    n134 = call "WaitForBuffer.vi"("ph"=w579, "sBufNr"=w570, "sBufNr 2"=w571, "timeout"=100, "error in (no error)"=w578) -> ("hout"=w581:u64)  [unwired: 10 in, 4 out]
                    n135 = call "GetImageBuffer2D.vi"("ph"=w581, "BuffIn"=w574, "BuffNr"=i16 0, "xRes"=w573, "yRes"=w572, "Bitresolution"=w567) -> ("BuffOut"=w565:u16[][])  [unwired: 6 in, 3 out]
                  }
                  frame #2 {
                    n136 = Quotient & Remainder(x=w608, y=u32 10) -> (floor(x/y)=w609:u32)  [unwired: 1 out]
                    n137 = Add(x=w609, y=w608) -> (x+y=w611:u32)
                    n138 = Wait (ms)(milliseconds to wait=w611) -> ()  [unwired: 1 out]
                  }
                  frame #3 {
                    w624 = 0
                    n139 = call <userlib>:"CameraGetData.vi"("Data Handle"=w633, "Camera Handle"=w637) -> ("Data Handle"=w632:u32)  [unwired: 1 in, 2 out]
                    n140 = call <userlib>:"DisplayImage.vi"("Image Handle"=w632, "Display Handle"=w634) -> ()  [unwired: 2 in, 2 out]
                    n141 = call <userlib>:"ImageGetArrayI32.vi"("Image Handle"=w632) -> ("Array int 32"=w630:i32[][])  [unwired: 2 in, 2 out]
                    n142 = To Word Integer(number=w630) -> (16bit integer=w629:i16[][])
                    n143 = Write to Binary File(file (use dialog)=w635, data=w629, 5:FALSE ("prepend array or string size? (T)"), 9:T5."little-endian" ("byte order (0:big-endian, network order)")) -> ()  [unwired: 2 in, 3 out]
                    n144 = Unbundle(w613) -> (w621:u16[][], "XResAct"=w620:u16, "YResAct"=w619:u16, "BufNrOut"=w618:i16, "BufNrOut"=w617:i16, "ErrorOut"=w616:errorcluster, "hout"=w615:u64, "Bits/pixel"=w614:u16)
                    n145 = call "AddBufferEX.vi"("ph"=w615, "BuffNr"=i16 0, "1stImage"=w624, "LastImage"=w624, "error in (no error)"=w616, "XRes"=w620, "YRes"=w619, "BitPerPixel"=w614) -> ("hout"=w626:u64, "error out"=w625:errorcluster)  [unwired: 5 in, 1 out]
                    n146 = call "WaitForBuffer.vi"("ph"=w626, "sBufNr"=w617, "sBufNr 2"=w618, "timeout"=100, "error in (no error)"=w625) -> ("hout"=w628:u64)  [unwired: 10 in, 4 out]
                    n147 = call "GetImageBuffer2D.vi"("ph"=w628, "BuffIn"=w621, "BuffNr"=i16 0, "xRes"=w620, "yRes"=w619, "Bitresolution"=w614) -> ("BuffOut"=w612:u16[][])  [unwired: 6 in, 3 out]
                  }
                  frame #4 {
                    n148 = Quotient & Remainder(x=w638, y=u32 10) -> (floor(x/y)=w639:u32)  [unwired: 1 out]
                    n149 = Add(x=w639, y=w638) -> (x+y=w641:u32)
                    n150 = Wait (ms)(milliseconds to wait=w641) -> ()  [unwired: 1 out]
                  }
                  frame #5 {
                    w654 = 0
                    n151 = call <userlib>:"CameraGetData.vi"("Data Handle"=w663, "Camera Handle"=w667) -> ("Data Handle"=w662:u32)  [unwired: 1 in, 2 out]
                    n152 = call <userlib>:"ImageGetArrayI32.vi"("Image Handle"=w662) -> ("Array int 32"=w660:i32[][])  [unwired: 2 in, 2 out]
                    n153 = call <userlib>:"DisplayImage.vi"("Image Handle"=w662, "Display Handle"=w664) -> ()  [unwired: 2 in, 2 out]
                    n154 = To Word Integer(number=w660) -> (16bit integer=w659:i16[][])
                    n155 = Write to Binary File(file (use dialog)=w665, data=w659, 5:FALSE ("prepend array or string size? (T)"), 9:T5."little-endian" ("byte order (0:big-endian, network order)")) -> ()  [unwired: 2 in, 3 out]
                    n156 = Unbundle(w643) -> (w651:u16[][], "XResAct"=w650:u16, "YResAct"=w649:u16, "BufNrOut"=w648:i16, "BufNrOut"=w647:i16, "ErrorOut"=w646:errorcluster, "hout"=w645:u64, "Bits/pixel"=w644:u16)
                    n157 = call "AddBufferEX.vi"("ph"=w645, "BuffNr"=i16 0, "1stImage"=w654, "LastImage"=w654, "error in (no error)"=w646, "XRes"=w650, "YRes"=w649, "BitPerPixel"=w644) -> ("hout"=w656:u64, "error out"=w655:errorcluster)  [unwired: 5 in, 1 out]
                    n158 = call "WaitForBuffer.vi"("ph"=w656, "sBufNr"=w647, "sBufNr 2"=w648, "timeout"=100, "error in (no error)"=w655) -> ("hout"=w658:u64)  [unwired: 10 in, 4 out]
                    n159 = call "GetImageBuffer2D.vi"("ph"=w658, "BuffIn"=w651, "BuffNr"=i16 0, "xRes"=w650, "yRes"=w649, "Bitresolution"=w644) -> ("BuffOut"=w642:u16[][])  [unwired: 6 in, 3 out]
                  }
                  frame #6 {
                    # "Indicate DB\nIssue"
                    # "Number of replacements is number of lines"
                    n160 = shared-variable-write(refnum<k21> "ni.var.psp://my computer/Untitled Library 1/CSHQ_1_Time" ("shared variable refnum in"), w673) -> ()  [unwired: 1 in, 2 out]
                    n161 = Search and Replace String(replace all?=TRUE ("replace all? (F)"), input string=w668, search string="(") -> (result string=w680:string)  [unwired: 5 in, 3 out]
                    n162 = Search and Replace String(replace all?=TRUE ("replace all? (F)"), input string=w680, search string=")") -> (result string=w672:string, number of replacements=w675:i32)  [unwired: 5 in, 2 out]
                    "Database Output" <- w672
                    n163 = String Length(string=w672) -> (length=w671:i32)
                    n164 = Greater?(x=w671, y=10) -> (0:w669:bool)
                    n165 = case shown="True" w669 {
                      frame False {
                        n166 = local write "Database OK?"(TRUE ("Database OK?")) -> ()
                      }
                      frame True {
                        "Database OK?" <- FALSE ("Database OK?")
                      }
                    }
                    n167 = for {
                      N: w675 -> [_]
                      tunnel: w672 -> [w703]
                      tunnel: w676 -> [w699]
                      i -> [w704]
                      w691 = T5."little-endian" ("byte order (0:big-endian, network order)")
                      n168 = Pick Line(multi-line string=w703, line index=w704) -> (output string=w702:string)  [unwired: 1 in]
                      n169 = Match Pattern(string=w702, regular expression="\\s") -> (before substring=w694:string, after substring=w700:string)  [unwired: 1 in, 2 out]
                      n170 = Fract/Exp String To Number(string=w700) -> (number=w688:dbl)  [unwired: 3 in, 1 out]
                      n171 = Concatenate Strings(w694) -> (w693:string)
                      n172 = To Double Precision Float(number=w688) -> (double precision float=w686:dbl)
                      n173 = Write to Binary File(file (use dialog)=w699, data=w693, 5:FALSE ("prepend array or string size? (T)"), 9:w691) -> (refnum out=w695:refnum<file>, error out=w696:errorcluster)  [unwired: 2 in, 1 out]
                      n174 = To Byte Integer(number=0) -> (8bit integer=w685:i8)
                      n175 = Write to Binary File(file (use dialog)=w695, data=w685, error in=w696, 5:FALSE ("prepend array or string size? (T)"), 9:T5."little-endian" ("byte order (0:big-endian, network order)")) -> (refnum out=w689:refnum<file>, error out=w692:errorcluster)  [unwired: 1 in, 1 out]
                      n176 = Write to Binary File(file (use dialog)=w689, data=w686, error in=w692, 5:FALSE ("prepend array or string size? (T)"), 9:w691) -> ()  [unwired: 1 in, 3 out]
                    }
                  }
                  frame #7 {
                    n177 = Close File(refnum=w705) -> ()  [unwired: 1 in, 2 out]
                  }
                }
                n178 = for {
                  N -> [w507]
                  shift-right: [w508] -> w433
                  shift-left: w434 -> [w510]
                  tunnel: w434 -> [w509] mode=indexing
                  i -> [w503]
                  n179 = Subtract(x=w507, y=1) -> (x-y=w505:i32)
                  n180 = Subtract(x=w505, y=w503) -> (x-y=w504:i32)
                  n181 = Replace Array Subset(array=w510, new element=w509, index (row)=w504) -> (w508:u16[][])  [unwired: 1 in]
                }
                n182 = Transpose 2D Array(2D array=w433) -> (transposed array=→"PF Atoms":u16[][])
                n183 = for {
                  N -> [w531]
                  shift-right: [w532] -> w442
                  shift-left: w443 -> [w534]
                  tunnel: w443 -> [w533] mode=indexing
                  i -> [w527]
                  n184 = Subtract(x=w531, y=1) -> (x-y=w529:i32)
                  n185 = Subtract(x=w529, y=w527) -> (x-y=w528:i32)
                  n186 = Replace Array Subset(array=w534, new element=w533, index (row)=w528) -> (w532:i16[][])  [unwired: 1 in]
                }
                n187 = for {
                  N -> [w499]
                  shift-right: [w500] -> w430
                  shift-left: w431 -> [w502]
                  tunnel: w431 -> [w501] mode=indexing
                  i -> [w495]
                  n188 = Subtract(x=w499, y=1) -> (x-y=w497:i32)
                  n189 = Subtract(x=w497, y=w495) -> (x-y=w496:i32)
                  n190 = Replace Array Subset(array=w502, new element=w501, index (row)=w496) -> (w500:u16[][])  [unwired: 1 in]
                }
                n191 = Transpose 2D Array(2D array=w442) -> (transposed array=→"Atoms":i16[][])
                n192 = Transpose 2D Array(2D array=w430) -> (transposed array=→"PF No Atoms":u16[][])
                n193 = Subtract(x=w443, y=w437) -> (x-y=w453:i16[][])
                n194 = for {
                  N -> [w491]
                  shift-right: [w492] -> w427
                  shift-left: w428 -> [w494]
                  tunnel: w428 -> [w493] mode=indexing
                  i -> [w487]
                  n195 = Subtract(x=w491, y=1) -> (x-y=w489:i32)
                  n196 = Subtract(x=w489, y=w487) -> (x-y=w488:i32)
                  n197 = Replace Array Subset(array=w494, new element=w493, index (row)=w488) -> (w492:u16[][])  [unwired: 1 in]
                }
                n198 = for {
                  N -> [w523]
                  shift-right: [w524] -> w440
                  shift-left: w438 -> [w526]
                  tunnel: w438 -> [w525] mode=indexing
                  i -> [w519]
                  n199 = Subtract(x=w523, y=1) -> (x-y=w521:i32)
                  n200 = Subtract(x=w521, y=w519) -> (x-y=w520:i32)
                  n201 = Replace Array Subset(array=w526, new element=w525, index (row)=w520) -> (w524:i16[][])  [unwired: 1 in]
                }
                n202 = Subtract(x=w438, y=w437) -> (x-y=w452:i16[][])
                n203 = Transpose 2D Array(2D array=w440) -> (transposed array=→"No Atoms":i16[][])
                n204 = Subtract(x=w431, y=w419) -> (x-y=w422:i32[][])
                n205 = Multiply(x=w422, y="PF Scale") -> (x*y=w421:dbl[][])
                n206 = Multiply(x=w452, y="Scaling") -> (x*y=w451:dbl[][])
                n207 = Subtract(x=w434, y=w419) -> (x-y=w420:i32[][])
                n208 = Divide(x=w420, y=w421) -> (x/y=w444:dbl[][])
                n209 = Divide(x=w453, y=w451) -> (x/y=w449:dbl[][])
                n210 = for {
                  N -> [w515]
                  shift-right: [w516] -> w436
                  shift-left: w437 -> [w518]
                  tunnel: w437 -> [w517] mode=indexing
                  i -> [w511]
                  n211 = Subtract(x=w515, y=1) -> (x-y=w513:i32)
                  n212 = Subtract(x=w513, y=w511) -> (x-y=w512:i32)
                  n213 = Replace Array Subset(array=w518, new element=w517, index (row)=w512) -> (w516:i16[][])  [unwired: 1 in]
                }
                n214 = for {
                  N -> [w540]
                  shift-right: [w541] -> w445
                  shift-left: w444 -> [w542]
                  tunnel: w444 -> [w535] mode=indexing
                  i -> [w536]
                  n215 = Subtract(x=w540, y=1) -> (x-y=w538:i32)
                  n216 = Subtract(x=w538, y=w536) -> (x-y=w537:i32)
                  n217 = Replace Array Subset(array=w542, new element=w535, index (row)=w537) -> (w541:dbl[][])  [unwired: 1 in]
                }
                n218 = Transpose 2D Array(2D array=w427) -> (transposed array=→"PF Dark":u16[][])
                n219 = Array Size(array=w449) -> ()  [unwired: 1 out]
                n220 = for {
                  N -> [w547]
                  shift-right: [w548] -> w450
                  shift-left: w449 -> [w550]
                  tunnel: w449 -> [w549] mode=indexing
                  i -> [w543]
                  n221 = Subtract(x=w547, y=1) -> (x-y=w545:i32)
                  n222 = Subtract(x=w545, y=w543) -> (x-y=w544:i32)
                  n223 = Replace Array Subset(array=w550, new element=w549, index (row)=w544) -> (w548:dbl[][])  [unwired: 1 in]
                }
                n224 = Transpose 2D Array(2D array=w436) -> (transposed array=→"Dark Field":i16[][])
                n225 = Get Queue Status(queue=w415) -> (queue out=w413:refnum<queue>, # elements in queue=w418:i32)  [unwired: 2 in, 6 out]
                n226 = Transpose 2D Array(2D array=w445) -> (transposed array=→"Intensity Graph":dbl[][])
                n227 = Less?(x=w418, y=5) -> (x < y?=w416:bool)
                n228 = Transpose 2D Array(2D array=w450) -> (transposed array=w414:dbl[][])
                n229 = case shown="False" w416 {
                  tunnel: w414 -> [w471 w486]
                  tunnel: w413 -> [w475 w485]
                  tunnel: [w467 w484] -> w412
                  frame False {
                    n230 = Flush Queue(queue=w475) -> (queue out=w473:refnum<queue>, remaining elements=w474:cluster{"Normalized Image":dbl[][]}[])  [unwired: 1 in, 1 out]
                    n231 = for {
                      tunnel: w474 -> [w483] mode=indexing
                      tunnel: w473 -> [w481]
                      tunnel: [w480] -> w472
                      n232 = Unbundle By Name(w483) -> ("Normalized Image"=w482:dbl[][])
                      n233 = Enqueue Element At Opposite End(queue=w481, element=w482) -> (queue out=w480:refnum<queue>)  [unwired: 2 in, 2 out]
                    }
                    n234 = Lossy Enqueue Element(queue=w472, element=w471) -> (queue out=w470:refnum<queue>)  [unwired: 1 in, 3 out]
                    n235 = Flush Queue(queue=w470) -> (queue out=w469:refnum<queue>, remaining elements=w468:cluster{"Normalized Image":dbl[][]}[])  [unwired: 1 in, 1 out]
                    n236 = for {
                      tunnel: w468 -> [w479] mode=indexing
                      tunnel: w469 -> [w477]
                      tunnel: [w476] -> w467
                      n237 = Unbundle By Name(w479) -> ("Normalized Image"=w478:dbl[][])
                      n238 = Enqueue Element At Opposite End(queue=w477, element=w478) -> (queue out=w476:refnum<queue>)  [unwired: 2 in, 2 out]
                    }
                  }
                  frame True {
                    n239 = Enqueue Element At Opposite End(queue=w485, element=w486) -> (queue out=w484:refnum<queue>)  [unwired: 2 in, 2 out]
                  }
                }
                n240 = shared-variable-write(refnum<k21> "ni.var.psp://my computer/Untitled Library 1/CSHQ_1_Changed" ("shared variable refnum in"), TRUE) -> ()  [unwired: 1 in, 2 out]
              }
            }
            n241 = Multiply(x=w295, y=1.021) -> (x*y=w293:dynamicdata)
            n242 = Add(x=-0.5356, y=w293) -> (x+y=→"Top of Chamber Monitor":dynamicdata)
            n243 = shared-variable-read(refnum<k21> "ni.var.psp://my computer/Untitled Library 1/CSHQ_1_Changed" ("shared variable refnum in"), TRUE) -> (w273:refnum<k21>, w266:bool)  [unwired: 1 in, 2 out]
            n244 = Get Queue Status(queue=w263) -> (queue out=w276:refnum<queue>, # elements in queue=w272:i32)  [unwired: 2 in, 6 out]
            n245 = case shown="True" w266 {
              tunnel: w273 -> [_ _]
              tunnel: w272 -> [_ w347]
              tunnel: w271 -> [w335 w348]
              tunnel: [w335 w346] -> w270
              tunnel: [TRUE w343] -> _
              tunnel: w263 -> [_ w337]
              frame False {
              }
              frame True {
                w343 = FALSE
                n246 = Less?(x=w347, y=5) -> (x < y?=w349:bool)
                n247 = case shown="True" w349 {
                  tunnel: w348 -> [w365 w400]
                  tunnel: w347 -> [_ w397]
                  tunnel: [w363 w398] -> w346
                  tunnel: [w362 w395] -> w338
                  frame False {
                    n248 = for {
                      N: 5 -> [_]
                      tunnel: w365 -> [w370]
                      shift-right: [w368] -> w363
                      shift-left: _ -> [w367]
                      tunnel: [w366] -> w362
                      i -> [w369]
                      w366 = 4.0 ("Value")
                      n249 = case shown="1..3" w369 {
                        selector: w369 -> [_ w379 w389]
                        tunnel: w370 -> [_ w380 w394]
                        tunnel: [cluster{"date/time string":string, i32}[] [] w378 w386] -> w368
                        tunnel: w367 -> [_ w377 w393]
                        frame 0, Default {
                        }
                        frame 1..3 {
                          n250 = Index Array(array=w380, index=w379) -> (element=w376:cluster{"date/time string":string, i32})
                          n251 = Unbundle(w376) -> ("date/time string"=w375:string, w374:i32)
                          n252 = Decrement(x=w374) -> (x-1=w373:i32)
                          n253 = Bundle("date/time string"=w375, w373) -> (w372:cluster{"date/time string":string, i32})  [unwired: 1 in]
                          n254 = Build Array (concatenate)(w377, w372) -> (w378:cluster{"date/time string":string, i32}[])
                        }
                        frame 4 {
                          n255 = Index Array(array=w394, index=w389) -> (element=w382:cluster{"date/time string":string, i32})
                          n256 = Unbundle(w382) -> ("date/time string"=w385:string, w384:i32)
                          n257 = Decrement(x=w384) -> (x-1=w383:i32)
                          n258 = Bundle("date/time string"=w385, w383) -> (w381:cluster{"date/time string":string, i32})  [unwired: 1 in]
                          n259 = Build Array (concatenate)(w393, w381) -> (w390:cluster{"date/time string":string, i32}[])
                          n260 = shared-variable-read(refnum<k21> "ni.var.psp://my computer/Untitled Library 1/CSHQ_1_Time" ("shared variable refnum in"), "bullshit" ("search string")) -> (w388:string)  [unwired: 1 in, 3 out]
                          n261 = Bundle("search string"=w388, w389) -> (w387:cluster{"search string":string, i32})  [unwired: 1 in]
                          n262 = Build Array (concatenate)(w390, w387) -> (w386:cluster{"search string":string, i32}[])
                        }
                      }
                      n263 = property on="Display Image" class="Ring (strict)"("Value"=w366) -> ()  [unwired: 2 in, 2 out]
                    }
                  }
                  frame True {
                    n264 = Subtract(x=w397, y=1) -> (x-y=w395:i32)
                    n265 = shared-variable-read(refnum<k21> "ni.var.psp://my computer/Untitled Library 1/CSHQ_1_Time" ("shared variable refnum in"), "string" ("search string")) -> (w401:string)  [unwired: 1 in, 3 out]
                    n266 = Bundle("search string"=w401, w395) -> (w399:cluster{"search string":string, i32})  [unwired: 1 in]
                    n267 = Build Array (concatenate)(w400, w399) -> (w398:cluster{"search string":string, i32}[])
                    n268 = property on="Display Image" class="Ring (strict)"("Value"=w395) -> ()  [unwired: 2 in, 2 out]
                  }
                }
                n269 = Wait (ms)(milliseconds to wait=u32 100) -> ()  [unwired: 1 out]
                n270 = Get Queue Status(queue=w337) -> (queue out=w336:refnum<queue>, # elements in queue=w342:i32)  [unwired: 2 in, 6 out]
                n271 = Flush Queue(queue=w336) -> (queue out=w340:refnum<queue>, remaining elements=w341:cluster{"Normalized Image":dbl[][]}[])  [unwired: 1 in, 1 out]
                n272 = To Word Integer(number=w338) -> (16bit integer=w339:i16)
                n273 = for {
                  tunnel: w341 -> [w360] mode=indexing
                  tunnel: w340 -> [w359]
                  tunnel: [w358] -> _
                  tunnel: w339 -> [w352]
                  tunnel: w342 -> [w353]
                  i -> [w357]
                  n274 = Increment(x=w352) -> (x+1=w351:i16)
                  n275 = Unbundle By Name(w360) -> ("Normalized Image"=w354:dbl[][])
                  n276 = Subtract(x=w353, y=w351) -> (x-y=w356:i32)
                  n277 = Equal?(x=w356, y=w357) -> (x = y?=w355:bool)
                  n278 = case shown="True" w355 {
                    tunnel: w354 -> [_ w361]
                    frame False {
                    }
                    frame True {
                      n279 = local write "Normalized Image"(w361) -> ()
                    }
                  }
                  n280 = Enqueue Element(queue=w359, element=w354) -> (queue out=w358:refnum<queue>)  [unwired: 2 in, 2 out]
                }
                n281 = shared-variable-write(refnum<k21> "ni.var.psp://my computer/Untitled Library 1/CSHQ_1_Changed" ("shared variable refnum in"), w343) -> ()  [unwired: 1 in, 2 out]
              }
            }
            n282 = Greater?(x=w272, y=0) -> (0:w268:bool)
            n283 = event shown="[0] Key Down;  \"Display Image\": Value Change" {
              selector: _ -> [_ _]
              dyn-events: _ -> [_ _]
              timeout: 1 -> [_ _]
              tunnel: [w313 w333] -> w277
              tunnel: w276 -> [w312 w333]
              tunnel: w272 -> [w311 _]
              tunnel: w268 -> [w310 _]
              tunnel: "Display Image" -> [w309 _]
              event Key Down; "Display Image": Value Change {
                n284 = event-data() -> ()  [unwired: 1 in, 2 out]
                n285 = case shown="True" w310 {
                  tunnel: [w314 w319] -> w313
                  tunnel: w312 -> [w314 w317]
                  tunnel: w311 -> [_ w316]
                  tunnel: w309 -> [_ w315]
                  frame False {
                  }
                  frame True {
                    n286 = Flush Queue(queue=w317) -> (queue out=w320:refnum<queue>, remaining elements=w321:cluster{"Normalized Image":dbl[][]}[])  [unwired: 1 in, 1 out]
                    n287 = To Word Integer(number=w315) -> (16bit integer=w318:i16)
                    n288 = for {
                      tunnel: w321 -> [w331] mode=indexing
                      tunnel: w320 -> [w330]
                      tunnel: [w329] -> w319
                      tunnel: w318 -> [w323]
                      tunnel: w316 -> [w324]
                      i -> [w328]
                      n289 = Increment(x=w323) -> (x+1=w322:i16)
                      n290 = Unbundle By Name(w331) -> ("Normalized Image"=w325:dbl[][])
                      n291 = Subtract(x=w324, y=w322) -> (x-y=w327:i32)
                      n292 = Equal?(x=w327, y=w328) -> (x = y?=w326:bool)
                      n293 = case shown="True" w326 {
                        tunnel: w325 -> [_ w332]
                        frame False {
                        }
                        frame True {
                          "Normalized Image" <- w332
                        }
                      }
                      n294 = Enqueue Element(queue=w330, element=w325) -> (queue out=w329:refnum<queue>)  [unwired: 2 in, 2 out]
                    }
                  }
                }
              }
              event Timeout {
                n295 = event-data() -> ()  [unwired: 1 in, 2 out]
              }
            }
            n296 = property on="Display Image" class="Ring (strict)"("StringsAndValues[]"=w270) -> ()  [unwired: 2 in, 2 out]
            n297 = Not(x="?") -> (.not. x?=w288:bool)
            n298 = And(x=w290, y=w288) -> (x .and. y?=w289:bool)
          }
        }
      }
      n299 = Wait (ms)(milliseconds to wait=u32 5) -> ()  [unwired: 1 out]
    }
    frame #3 {
      w712 = u16 0 items=["Stop", "Run"] ("RecordingState")
      # "CoolSnapHQ"
      # "Stop recording"
      # "Step 3:\nClose the handles."
      n300 = call "CancelImages.vi"("ph"=w711) -> ("error out"=w714:errorcluster, "hout"=w713:u64)  [unwired: 2 in, 1 out]
      n301 = call "SetRecordingState.vi"("ErrorIn"=w714, "RecordingState"=w712, "ph"=w713) -> ("ErrorOut"=w706:errorcluster, "hout"=w707:u64)  [unwired: 2 in, 1 out]
      n302 = call "ExSubCloseExperimentCoolSnap.vi"("Handles In"=w715) -> ()  [unwired: 1 in, 1 out]
      n303 = call "Cleanup.vi"("error in (no error)"=w706, "ph"=w707) -> ("error out"=w709:errorcluster, "hout"=w708:u64)  [unwired: 8 in]
      n304 = call "CloseCamera.vi"("ErrorIn"=w709, "Handle in"=w708) -> ("ErrorOut"=w710:errorcluster)  [unwired: 1 in, 2 out]
      n305 = call <vilib>:"Simple Error Handler.vi"("error in (no error)"=w710) -> ()  [unwired: 4 in, 5 out]
    }
  }
